vi "create.vi"(8 "error in (no error)":errorcluster) -> (0 "error out":errorcluster, 3 "OSA300 out":refnum<class "OSA300.lvclass">)   [LabVIEW 2010, in "OSA300.lvclass"]
uses:
  OSA300.lvclass
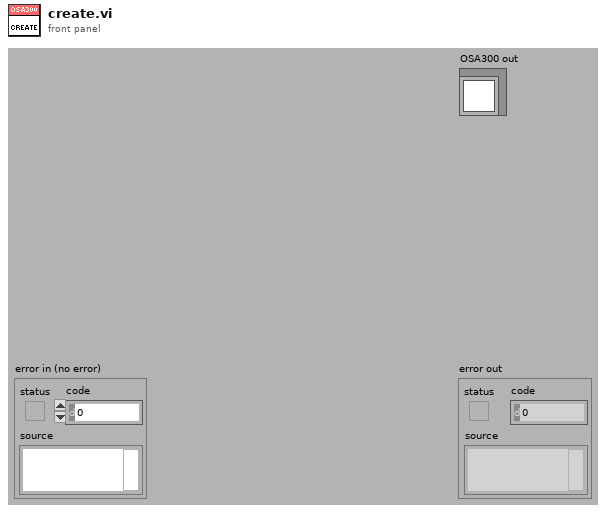
[diagram p1: front panel]
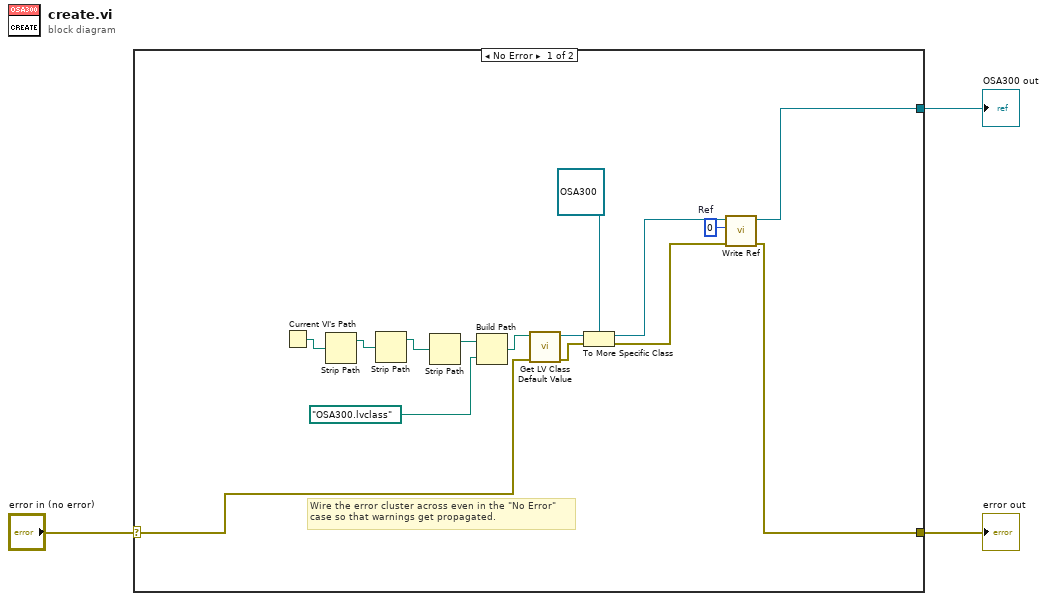
[diagram p0: block diagram]
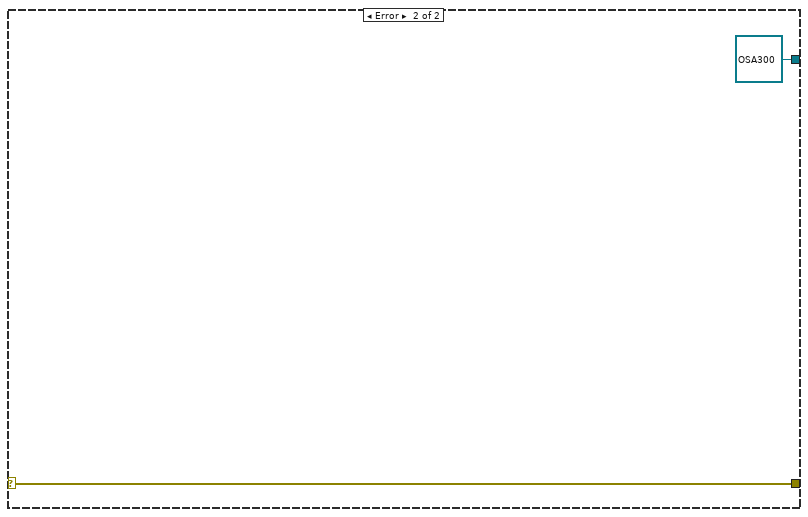
[diagram p2: hidden frame]
diagram:
  n1 = case shown="No Error" "error in (no error)" {
    selector: "error in (no error)" -> [w10 w20]
    tunnel: [w8 w20] -> w2
    tunnel: [w7 refnum<class "OSA300.lvclass"> refnum ("OSA300 out")] -> w1
    frame No Error {
      w5 = u32 0  # Ref
      # "Wire the error cluster across even in the \"No Error\"\ncase so that warnings get propagated."
      n2 = Current VI's Path() -> (path=w18:path)
      n3 = Strip Path(path=w18) -> (stripped path=w17:path)  [unwired: 1 out]
      n4 = Strip Path(path=w17) -> (stripped path=w16:path)  [unwired: 1 out]
      n5 = Strip Path(path=w16) -> (stripped path=w15:path)  [unwired: 1 out]
      n6 = Build Path(base path=w15, name or relative path=path "OSA300.lvclass") -> (appended path=w14:path)
      n7 = call <vilib>:"Get LV Class Default Value.vi"("error in (no error)"=w10, "class path"=w14) -> ("error out"=w11:errorcluster, "object"=w12:refnum<class>)  [unwired: 8 in]
      n8 = To More Specific Class(target class=refnum<class "OSA300.lvclass"> refnum ("OSA300 out"), reference=w12, error in=w11) -> (specific class reference=w6:refnum<class "OSA300.lvclass">, error out=w9:errorcluster)
      n9 = call "Write Ref.vi"("error in (no error)"=w9, "Ref"=w5, "OSA300 in"=w6) -> ("error out"=w8:errorcluster, "OSA300 out"=w7:refnum<class "OSA300.lvclass">)  [unwired: 7 in]
    }
    frame Error {
    }
  }
  "error out" <- w2
  "OSA300 out" <- w1
